vi "Get Status.vi"(8 "error in (no error)":errorcluster, 11 "MSOX6004 in":refnum<class "MSOX6004.lvclass">) -> (0 "error out":errorcluster, 2 "Status Array":bool[](array[boolean]), 3 "MSOX6004 out":refnum<class "MSOX6004.lvclass">)   [LabVIEW 2018, in "MSOX6004.lvlib" / "MSOX6004.lvclass"]
doc: "This Override method is used to get the Oscope instrument status. The status data MUST be formatted into the 'Status Array' indicator as 1D array of boolean data ."
uses:
  MSOX6004.lvclass
  MSOX6004.lvclass/MSOX6004.ctl
  <instrlib>/Keysight InfiniiVision/Keysight InfiniiVision.lvlib
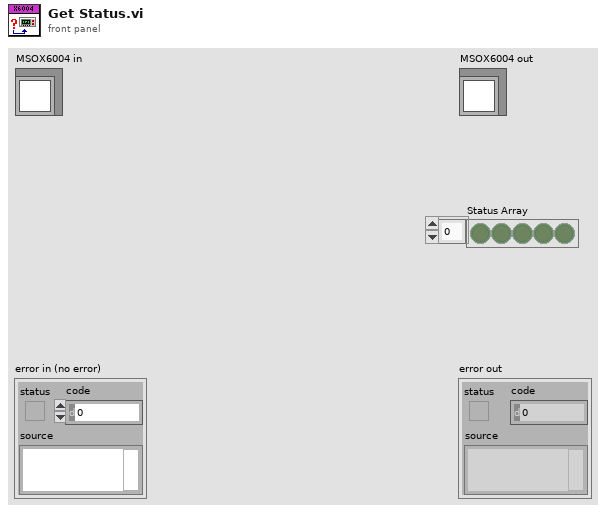
[diagram p1: front panel]
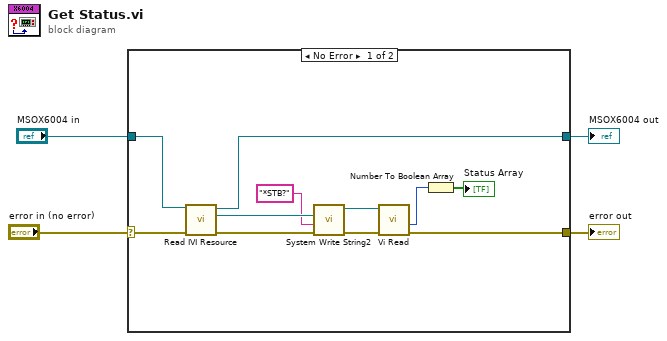
[diagram p0: block diagram]
diagram:
  n1 = case shown="No Error" "error in (no error)" {
    selector: "error in (no error)" -> [w15 w16]
    tunnel: "MSOX6004 in" -> [w14 w17]
    tunnel: [w5 w17] -> w2
    tunnel: [w8 w16] -> w1
    frame No Error {
      n2 = call "Read IVI Resource.vi"("error in (no error)"=w15, "MSOX6004 in"=w14) -> ("error out"=w12:errorcluster, "IVI Resource"=w13:refnum<k15>, "MSOX6004 out"=w5:refnum<class "MSOX6004.lvclass">)  [unwired: 7 in]
      n3 = call <instrlib>:"System Write String2.vi"("error in (no error)"=w12, "Data"="*STB?", "instrument handle"=w13) -> ("error out"=w9:errorcluster, "instrument handle out"=w10:refnum<k15>)  [unwired: 7 in]
      n4 = call <instrlib>:"Vi Read.vi"("error in (no error)"=w9, "instrument handle"=w10) -> ("error out"=w8:errorcluster, "ReturnCount"=w7:i64)  [unwired: 6 in, 2 out]
      n5 = Number To Boolean Array(number=w7) -> (Boolean array=→"Status Array":bool[])
    }
    frame Error {
    }
  }
  "error out" <- w1
  "MSOX6004 out" <- w2
